vi "IV Sweep.vi"(0 "Resource":refnum<k15>="4139_1", 1 "Pulse On Time (s)":dbl(slide)=5e-05 scale=1e-05..0.01 scale format="%#_2p", 5 "Source Delay":dbl=1e-05 format="%_3p", 7 "Aperture Time":dbl=3e-05 caption="Sample Rate" format="%_3p", 9 "# Samples":i32=500, 11 "Error In":errorcluster) -> (6 "XY Graph":T1(graph), 15 "Error Out":errorcluster)   [LabVIEW 2014]
doc: "Desmonstrates how to use the DCPower Pulse API to generate a Voltage or Current Pulse Sequence. This example initializes a session, configures the Source Mode and the Output Function, configures the pulse parameters, initiates the pulse output sequence, and takes measurements. The Tab Control on the front panel determines whether the example generates a voltage or current pulse sequence."
uses:
  <instrlib>/niDCPower/nidcpower.llb/niDCPower Source Mode.ctl
  <instrlib>/niDCPower/nidcpower.llb/niDCPower Output Function.ctl
  <instrlib>/niDCPower/nidcpower.llb/niDCPower Sequence Attribute Type.ctl
  <vilib>/Analysis/1siggen.llb/Ramp Pattern by Samples.vi
  <vilib>/Utility/file.llb/Write To Spreadsheet File (DBL).vi
  <vilib>/Analysis/NI_AALBase.lvlib
panel:
  in  "Transient Response Parameters":T2={"Gain Bandwidth"=280000.0, "Compensation Frequency"=225000.0, "Pole Zero Ratio"=2.1, "Gain Bandwidth V"=44500.0, "Compensation Frequency V"=8700.0, "Pole Zero Ratio V"=1.0}
  in  "Gain Bandwidth V":dbl(slide)=44500.0 scale=10.0..5000000.0 scale format="%#_6p"
  in  "Pole Zero Ratio V":dbl(slide)=1.0 scale=0.2..8.0
  in  "Compensation Frequency V":dbl(slide)=8700.0 scale=50.0..300000.0 scale format="%#_6p"
  in  "Compensation Frequency":dbl(slide)=225000.0 scale=50.0..300000.0 scale format="%#_6p"
  in  "Pole Zero Ratio":dbl(slide)=2.1 scale=0.2..8.0
  in  "Gain Bandwidth":dbl(slide)=280000.0 scale=10.0..5000000.0 scale format="%#_6p"
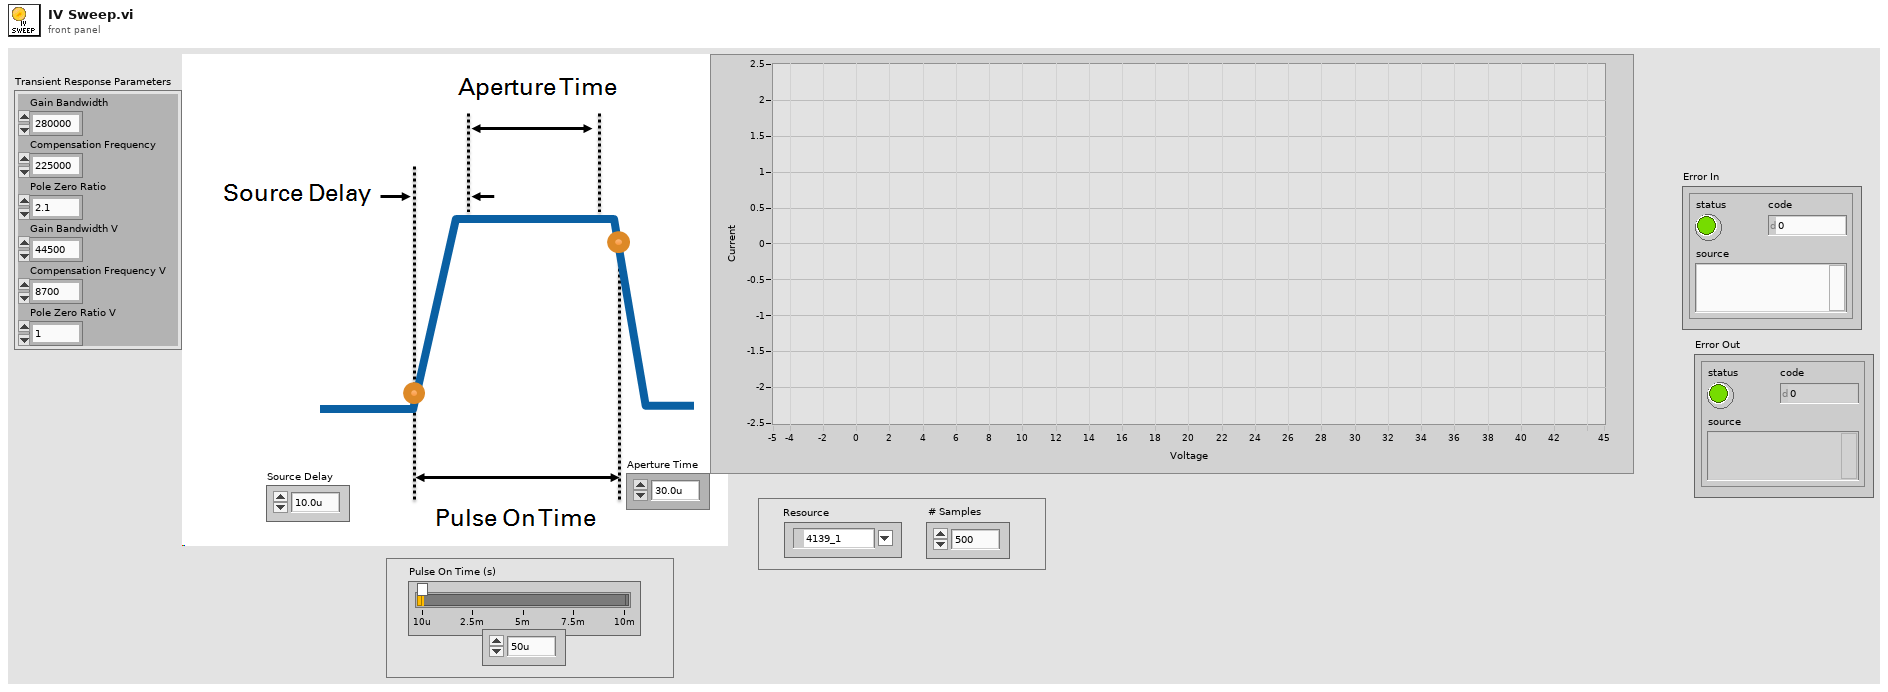
[diagram p1: front panel]
types:
  T1 = cluster{"voltage measurements":dbl[], "current measurements":dbl[]}
  T2 = cluster{"Gain Bandwidth":dbl, "Compensation Frequency":dbl, "Pole Zero Ratio":dbl, "Gain Bandwidth V":dbl, "Compensation Frequency V":dbl, "Pole Zero Ratio V":dbl}
  T3 = typedef "niDCPower Sequence Attribute Type.ctl" = i32
  T4 = typedef "niDCPower Output Function.ctl" = i32
  T5 = typedef "niDCPower Source Mode.ctl" = i32
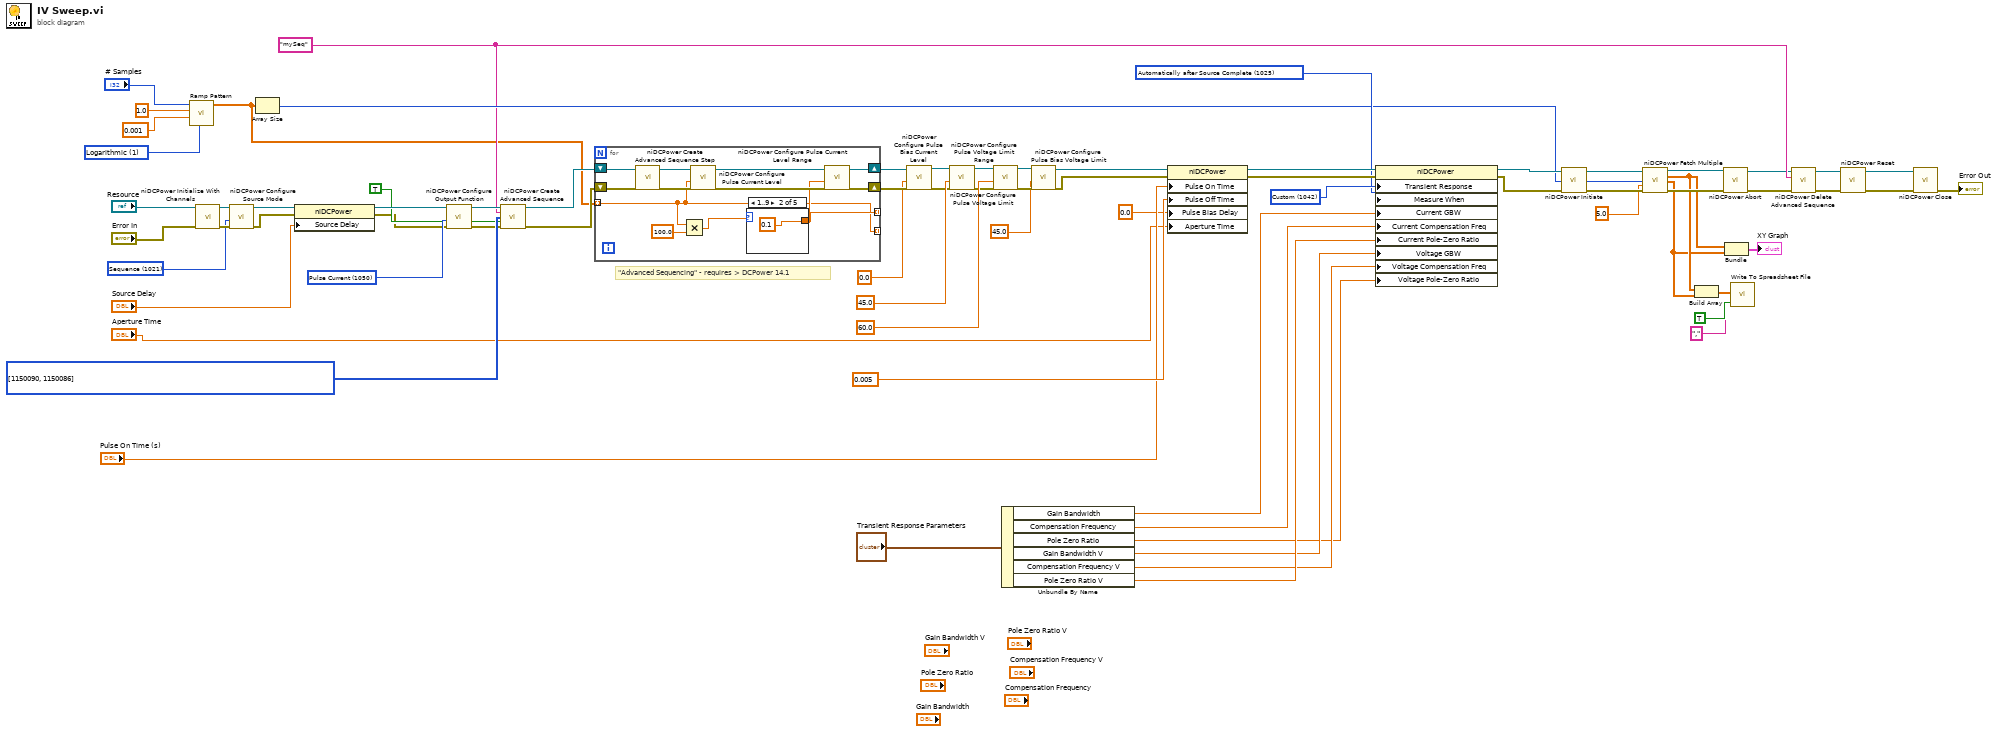
[diagram p0: block diagram]
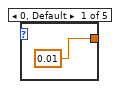
[diagram p2: hidden frame]
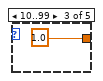
[diagram p3: hidden frame]
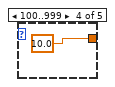
[diagram p4: hidden frame]
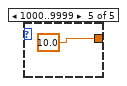
[diagram p5: hidden frame]
diagram:
  w32 = T3[] [1150090, 1150086] items=["Source -> Output Function"=1150008, "Source -> Output Enabled"=1250006, "Source -> Output Resistance"=1150061, "Source -> Transient Response"=1150062, "Source -> Custom Transient Response -> Voltage Gain Bandwidth"=1150067, "Source -> Custom Transient Response -> Voltage Compensation Frequency"=1150068, "Source -> Custom Transient Response -> Voltage Pole-Zero Ratio"=1150069, "Source -> Custom Transient Response -> Current Gain Bandwidth"=1150070, "Source -> Custom Transient Response -> Current Compensation Frequency"=1150071, "Source -> Custom Transient Response -> Current Pole-Zero Ratio"=1150072, "Source -> DC Voltage -> Voltage Level"=1250001, "Source -> DC Voltage -> Voltage Level Range"=1150005, "Source -> DC Voltage -> Current Limit"=1250005, "Source -> DC Voltage -> Current Limit Range"=1150004, "Source -> DC Current -> Current Level"=1150009, "Source -> DC Current -> Current Level Range"=1150011, "Source -> DC Current -> Voltage Limit"=1150010, "Source -> DC Current -> Voltage Limit Range"=1150012, "Source -> Pulse Voltage -> Pulse Voltage Level"=1150080, "Source -> Pulse Voltage -> Pulse Bias Voltage Level"=1150082, "Source -> Pulse Voltage -> Pulse Voltage Level Range"=1150084, "Source -> Pulse Voltage -> Pulse Current Limit"=1150081, "Source -> Pulse Voltage -> Pulse Bias Current Limit"=1150083, "Source -> Pulse Voltage -> Pulse Current Limit Range"=1150085, "Source -> Pulse Current -> Pulse Current Level"=1150086, "Source -> Pulse Current -> Pulse Bias Current Level"=1150088, "Source -> Pulse Current -> Pulse Current Level Range"=1150090, "Source -> Pulse Current -> Pulse Voltage Limit"=1150087, "Source -> Pulse Current -> Pulse Bias Voltage Limit"=1150089, "Source -> Pulse Current -> Pulse Voltage Limit Range"=1150091, "Source -> Advanced -> Source Delay"=1150051, "Source -> Advanced -> Pulse Bias Delay"=1150092, "Source -> Advanced -> Pulse On Time"=1150093, "Source -> Advanced -> Pulse Off Time"=1150094, "Measurement -> Sense"=1150013, "Measurement -> Aperture Time"=1150058, "Measurement -> Measure Record Length"=1150063, "Measurement -> Advanced -> DC Noise Rejection"=1150066] ("advanced sequence properties")
  w27 = "mySeq" ("sequence name")
  w34 = u16 1 items=["Linear", "Logarithmic"] ("type")
  w65 = 1042 items=["Slow"=1041, "Normal"=1038, "Fast"=1039, "Custom"=1042] ("Transient Response")
  w43 = T4 1050 items=["DC Voltage"=1006, "DC Current"=1007, "Pulse Voltage"=1049, "Pulse Current"=1050] ("output function")
  w64 = 1025 items=["Automatically after Source Complete"=1025, "On Demand"=1026, "On Measure Trigger"=1027] ("Measurement:Advanced:Measure When")
  w72 = T5 1021 items=["Single Point"=1020, "Sequence"=1021] ("source mode")
  # "\"Advanced Sequencing\" - requires > DCPower 14.1"
  n1 = call-poly <vilib>:"Ramp Pattern.vi"("type"=w34, "start"=0.001 ("Sweep Start"), "end"=1.0 ("Sweep End"), "samples"="# Samples") -> ("Ramp Pattern"=w25:dbl[])  [unwired: 6 in, 1 out]
  n2 = call <instrlib>:"niDCPower Initialize With Channels.vi"("error in (no error)"="Error In", "resource name"="Resource") -> ("error out"=w73:errorcluster, "instrument handle out"=w71:refnum<k15>)  [unwired: 2 in, 6 out]
  n3 = call <instrlib>:"niDCPower Configure Source Mode.vi"("error in (no error)"=w73, "source mode"=w72, "instrument handle"=w71) -> ("error out"=w24:errorcluster, "instrument handle out"=w22:refnum<k15>)  [unwired: 7 out]
  n4 = Array Size(array=w25) -> (size(s)=w52:i32)
  n5 = property class="niDCPower"(reference=w22, error in=w24, "Source Delay"="Source Delay") -> (reference out=w21:refnum<k15>, error out=w23:errorcluster)
  n6 = call <instrlib>:"niDCPower Configure Output Function.vi"("error in (no error)"=w23, "output function"=w43, "instrument handle"=w21) -> ("error out"=w31:errorcluster, "instrument handle out"=w33:refnum<k15>)  [unwired: 1 in, 6 out]
  n7 = call <instrlib>:"niDCPower Create Advanced Sequence.vi"("instrument handle"=w33, "sequence name"=w27, "advanced sequence properties"=w32, "set as active sequence"=TRUE, "error in (no error)"=w31) -> ("instrument handle out"=w29:refnum<k15>, "error out"=w30:errorcluster)  [unwired: 9 in]
  n8 = for {
    shift-right: [w84] -> w51
    shift-left: w30 -> [w78]
    shift-right: [w83] -> w50
    shift-left: w29 -> [w80]
    tunnel: w25 -> [w75] mode=indexing
    tunnel: [w75] -> _ mode=indexing
    tunnel: [w76] -> _ mode=indexing
    n9 = call <instrlib>:"niDCPower Create Advanced Sequence Step.vi"("error in (no error)"=w78, "instrument handle"=w80) -> ("error out"=w77:errorcluster, "instrument handle out"=w79:refnum<k15>)  [unwired: 8 in]
    n10 = Multiply(x=w75, y=100.0) -> (x*y=w74:dbl)
    n11 = call <instrlib>:"niDCPower Configure Pulse Current Level.vi"("error in (no error)"=w77, "pulse current level"=w75, "instrument handle"=w79) -> ("error out"=w82:errorcluster, "instrument handle out"=w81:refnum<k15>)  [unwired: 7 in]
    n12 = case shown="1..9" w74 {
      tunnel: [0.01 ("y") 0.1 ("y") 1.0 ("y") 10.0 ("y") 10.0 ("y")] -> w76
      frame 0, Default {
      }
      frame 1..9 {
      }
      frame 10..99 {
      }
      frame 100..999 {
      }
      frame 1000..9999 {
      }
    }
    n13 = call <instrlib>:"niDCPower Configure Pulse Current Level Range.vi"("error in (no error)"=w82, "pulse current level range"=w76, "instrument handle"=w81) -> ("error out"=w84:errorcluster, "instrument handle out"=w83:refnum<k15>)  [unwired: 7 in]
  }
  n14 = call <instrlib>:"niDCPower Configure Pulse Bias Current Level.vi"("error in (no error)"=w51, "pulse bias current level"=0.0 ("Pulse Bias Current Level"), "instrument handle"=w50) -> ("error out"=w49:errorcluster, "instrument handle out"=w48:refnum<k15>)  [unwired: 7 in]
  n15 = call <instrlib>:"niDCPower Configure Pulse Voltage Limit.vi"("error in (no error)"=w49, "pulse voltage limit"=45.0 ("Voltage Limit"), "instrument handle"=w48) -> ("error out"=w47:errorcluster, "instrument handle out"=w46:refnum<k15>)  [unwired: 7 in]
  n16 = call <instrlib>:"niDCPower Configure Pulse Voltage Limit Range.vi"("error in (no error)"=w47, "pulse voltage limit range"=60.0 ("Voltage Limit Range"), "instrument handle"=w46) -> ("error out"=w45:errorcluster, "instrument handle out"=w44:refnum<k15>)  [unwired: 7 in]
  n17 = Unbundle By Name("Transient Response Parameters") -> ("Gain Bandwidth"=w11:dbl, "Compensation Frequency"=w10:dbl, "Pole Zero Ratio"=w6:dbl, "Gain Bandwidth V"=w8:dbl, "Compensation Frequency V"=w7:dbl, "Pole Zero Ratio V"=w9:dbl)
  n18 = call <instrlib>:"niDCPower Configure Pulse Bias Voltage Limit.vi"("error in (no error)"=w45, "pulse bias voltage limit"=45.0 ("Pulse Bias Voltage Limit"), "instrument handle"=w44) -> ("error out"=w42:errorcluster, "instrument handle out"=w41:refnum<k15>)  [unwired: 7 in]
  n19 = property class="niDCPower"(reference=w41, error in=w42, "Pulse On Time"="Pulse On Time (s)", "Pulse Off Time"=0.005 ("Pulse Off Time (s)"), "Pulse Bias Delay"=0.0 ("Source:Advanced:Pulse Bias Delay"), "Aperture Time"="Aperture Time") -> (reference out=w70:refnum<k15>, error out=w69:errorcluster)
  n20 = property class="niDCPower"(reference=w70, error in=w69, "Transient Response"=w65, "Measure When"=w64, "Current GBW"=w11, "Current Compensation Freq"=w10, "Current Pole-Zero Ratio"=w9, "Voltage GBW"=w8, "Voltage Compensation Freq"=w7, "Voltage Pole-Zero Ratio"=w6) -> (reference out=w62:refnum<k15>, error out=w63:errorcluster)
  n21 = call <instrlib>:"niDCPower Initiate.vi"("error in (no error)"=w63, "instrument handle"=w62) -> ("error out"=w66:errorcluster, "instrument handle out"=w67:refnum<k15>)  [unwired: 2 in, 6 out]
  n22 = call <instrlib>:"niDCPower Fetch Multiple.vi"("instrument handle"=w67, "count (1)"=w52, "timeout (sec)"=5.0, "error in (no error)"=w66) -> ("instrument handle out"=w19:refnum<k15>, "voltage measurements"=w5:dbl[], "current measurements"=w4:dbl[], "error out"=w17:errorcluster)  [unwired: 6 in, 2 out]
  n23 = Build Array(w5, w4) -> (w3:dbl[][])
  n24 = call <instrlib>:"niDCPower Abort.vi"("error in (no error)"=w17, "instrument handle"=w19) -> ("error out"=w16:errorcluster, "instrument handle out"=w18:refnum<k15>)  [unwired: 8 in]
  n25 = Bundle("voltage measurements"=w5, "current measurements"=w4) -> (→"XY Graph":T1)  [unwired: 1 in]
  n26 = call-poly <vilib>:"Write To Spreadsheet File.vi"("delimiter (\\t)"="," ("delimiter (\\t)"), "transpose? (no:F)"=TRUE, "2D data"=w3) -> ()  [unwired: 5 in, 1 out]
  n27 = call <instrlib>:"niDCPower Delete Advanced Sequence.vi"("error in (no error)"=w16, "sequence name"=w27, "instrument handle"=w18) -> ("error out"=w15:errorcluster, "instrument handle out"=w14:refnum<k15>)  [unwired: 7 in]
  n28 = call <instrlib>:"niDCPower Reset.vi"("error in (no error)"=w15, "instrument handle"=w14) -> ("error out"=w54:errorcluster, "instrument handle out"=w53:refnum<k15>)  [unwired: 8 in]
  n29 = call <instrlib>:"niDCPower Close.vi"("error in (no error)"=w54, "instrument handle"=w53) -> ("error out"=→"Error Out":errorcluster)  [unwired: 9 out]
